vi "get_content.vi"(8 "error in (no error)":errorcluster, 11 "IDocument in":refnum<class "IReport.lvclass">) -> (0 "error out":errorcluster, 2 "String":string, 3 "IDocument out":refnum<class "IReport.lvclass">)   [LabVIEW 2024, in "IReport.lvclass"]
uses:
  IReport.lvclass
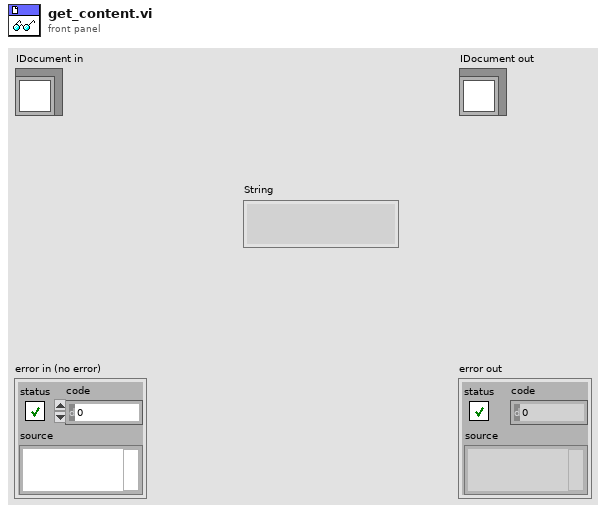
[diagram p1: front panel]
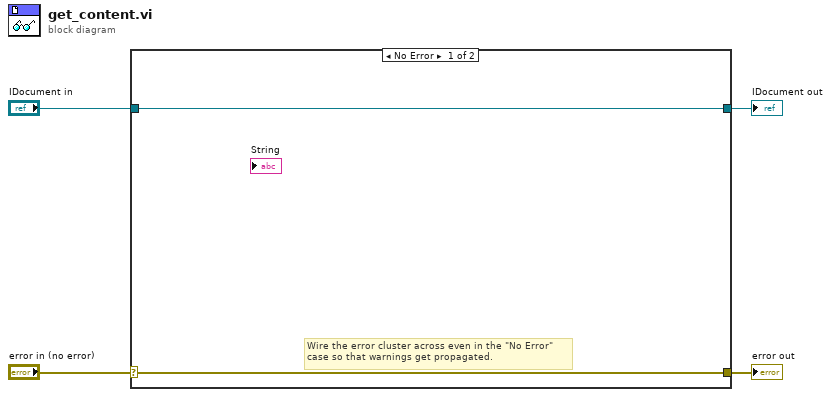
[diagram p0: block diagram]
diagram:
  n1 = case shown="No Error" "error in (no error)" {
    selector: "error in (no error)" -> [w5 w8]
    tunnel: [w5 w8] -> w3
    tunnel: [w6 w7] -> w1
    tunnel: "IDocument in" -> [w6 w7]
    frame No Error {
      # "Wire the error cluster across even in the \"No Error\"\ncase so that warnings get propagated."
    }
    frame Error {
    }
  }
  "error out" <- w3
  "IDocument out" <- w1
